vi "题目2.vi"() -> ()   [LabVIEW 2017]
panel:
  out "和2":dbl
  out "和":dbl
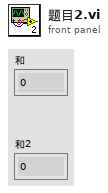
[diagram p1: front panel]
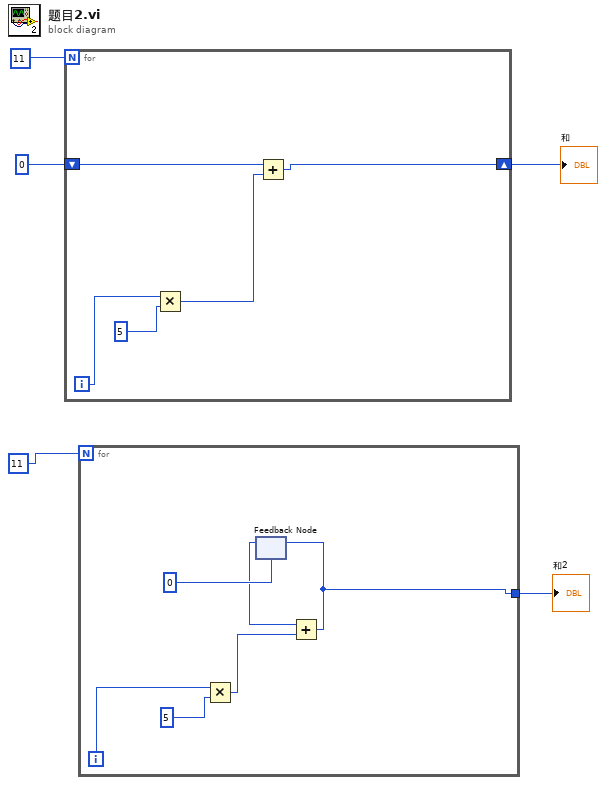
[diagram p0: block diagram]
diagram:
  n1 = for {
    N: 11 -> [_]
    shift-right: [w6] -> w3
    shift-left: 0 -> [w8]
    i -> [w10]
    n2 = Multiply(x=w10, y=5) -> (x*y=w7:i32)
    n3 = Add(x=w8, y=w7) -> (x+y=w6:i32)
  }
  "和" <- w3
  n4 = for {
    N: 11 -> [_]
    tunnel: [w11] -> w1
    i -> [w15]
    n5 = Multiply(x=w15, y=5) -> (x*y=w12:i32)
    n6 = feedback #1(0) -> (w13:i32)
    n7 = Add(x=w13, y=w12) -> (x+y=w11:i32)
    n8 = feedback-in #1(w11) -> ()
  }
  "和2" <- w1
